vi "Lookup Beacon Info From BT Address.vi"(11 "BT Address":string) -> (0 "found?":bool, 1 "Minor":string, 2 "Major":string, 3 "UUID":string)   [LabVIEW 2013]
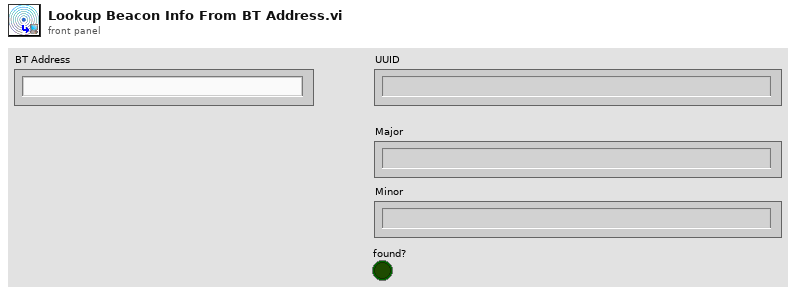
[diagram p1: front panel]
types:
  T1 = typedef "JSON Key List.ctl" = cluster{"X-M2X-KEY":string, "M2X Feed ID":string, "Twitter Access Token":string, "Twitter Access Secret":string, "Twitter Client Token":string, "Twitter Client Secret":string, "NTP Server":string, "Beacons":cluster{"UUID":string, "Major":string, "Minor":string, "BT Address":string}[], "Mic Stream":string}
  T2 = cluster{"UUID":string, "Major":string, "Minor":string, "BT Address":string}[]
  T3 = cluster{"UUID":string, "Major":string, "Minor":string, "BT Address":string}
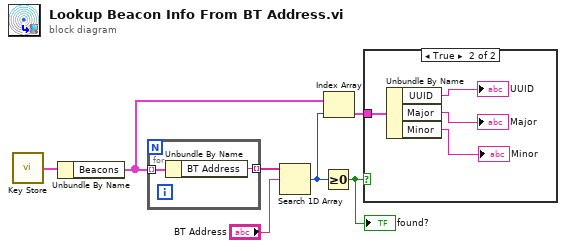
[diagram p0: block diagram]
diagram:
  n1 = call "Key Store.vi"() -> ("Current Store"=w7:T1)  [unwired: 1 in]
  n2 = Unbundle By Name(w7) -> ("Beacons"=w2:T2)
  n3 = for {
    tunnel: w2 -> [w9] mode=indexing
    tunnel: [w8] -> w6 mode=indexing
    n4 = Unbundle By Name(w9) -> ("BT Address"=w8:string)
  }
  n5 = Search 1D Array(1D array=w6, element="BT Address") -> (index of element=w3:i32)  [unwired: 1 in]
  n6 = Greater Or Equal To 0?(x=w3) -> (x >= 0?=w4:bool)
  "found?" <- w4
  n7 = Index Array(array=w2, index=w3) -> (element=w1:T3)
  n8 = case shown="True" w4 {
    tunnel: w1 -> [_ w13]
    frame False {
    }
    frame True {
      n9 = Unbundle By Name(w13) -> ("UUID"=→"UUID":string, "Major"=→"Major":string, "Minor"=→"Minor":string)
    }
  }
